vi "Process each eye.vi"(0 "Camera coordinates rel to head co-ordinates":T1 {"y" format="%.2f"; "z" format="%.2f"; "theta" format="%.2f"; "phi" format="%.2f"; "d" format="%.2f"}, 1 "Time (sec)":sgl[](array[numeric]) format="%.4f", 2 "Dir":enum16{"Right", "Left"}(ring), 3 "Hor (F)":dbl[](array[numeric]) format="%.2f", 4 "Ver (F)":dbl[](array[numeric]) format="%.2f", 5 "Posn, Vel, Acc 2":dbl[][](array[numeric]), 6 "Angles":bool, 7 "Point1":dbl[][](array[numeric]) format="%.2f", 8 "Trigger Edge":i32, 9 "Tor (F)":dbl[](array[numeric]) format="%.2f", 10 "Position Convention":u16(ring) items=["Fick Angles", "Rotation Vectors"], 11 "Point2":dbl[][](array[numeric]) format="%.2f", 12 "Sample Rate":i32, 13 "Point3":dbl[][](array[numeric]) format="%.2f", 16 "Savol Filter in percent":dbl=3.0 format="%#_13g", 18 "Use Last":bool, 19 "VOG system":enum16{"Mouse", "Chinchilla"}(ring)) -> (14 "Posn, Vel, Acc":dbl[][](array[numeric]) format="%.2f", 17 "cancelled":bool)   [LabVIEW 2016, in "3 dot tracker.lvlib"]
uses:
  3 dot tracker.lvlib
  <vilib>/Analysis/3filter.llb/Savitzky-Golay Filter (DBL).vi
  <vilib>/Analysis/baseanly.llb/A x Vector.vi
  comm/fick-matrix/fick-matrix.lvlib
  <vilib>/Analysis/NI_AALBase.lvlib
  comm/quaternion/quaternion.lvlib
  <vilib>/ptbypt/NI_PtbyPt.lvlib
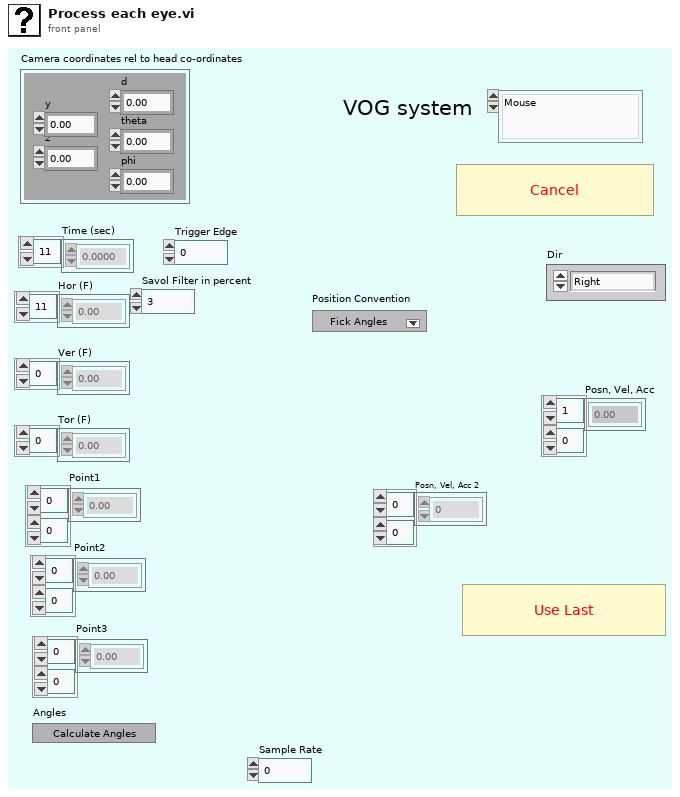
[diagram p1: front panel]
types:
  T1 = cluster{"d":dbl, "phi":dbl, "theta":dbl, "z":dbl, "y":dbl}
  T2 = cluster{"Point1":dbl[], "Point2":dbl[], "Point3":dbl[]}
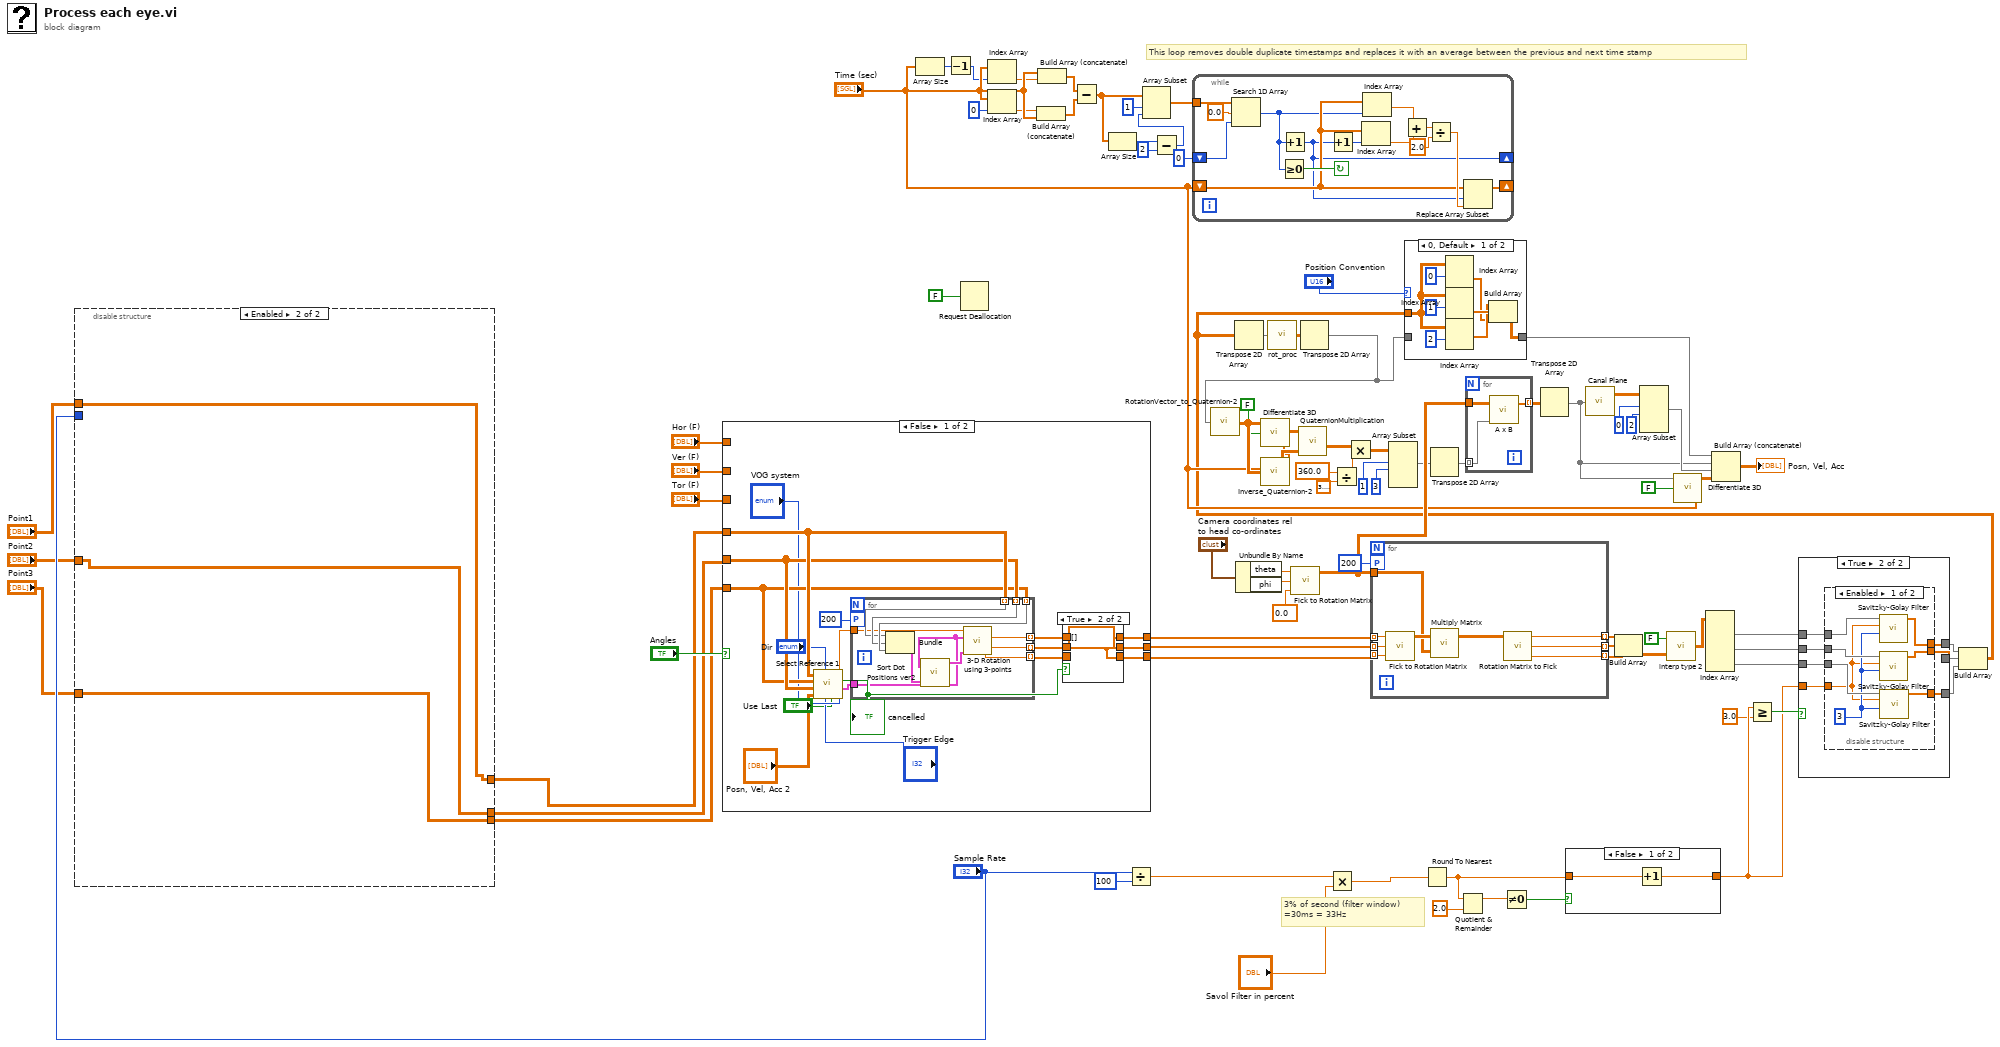
[diagram p0: block diagram]
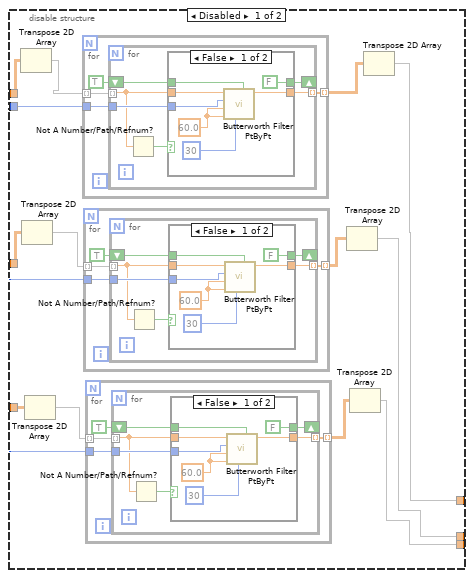
[diagram p2: hidden frame]
diagram:
  # "3% of second (filter window)\n=30ms = 33Hz"
  # "This loop removes double duplicate timestamps and replaces it with an average between the previous and next time stamp"
  n1 = disable-structure shown="Enabled" {
    disable-tunnel: "Sample Rate" -> [w100 _]
    disable-tunnel: "Point1" -> [w99 w160]
    disable-tunnel: [w96 w160] -> w5
    disable-tunnel: [w94 w158] -> w4
    disable-tunnel: [w93 w159] -> w3
    disable-tunnel: "Point2" -> [w90 w159]
    disable-tunnel: "Point3" -> [w89 w158]
    frame Disabled {
      n2 = Transpose 2D Array(2D array=w99) -> (transposed array=w98:dbl[][])
      n3 = Transpose 2D Array(2D array=w90) -> (transposed array=w91:dbl[][])
      n4 = Transpose 2D Array(2D array=w89) -> (transposed array=w88:dbl[][])
      n5 = for {
        tunnel: w98 -> [w142] mode=indexing
        tunnel: w100 -> [w141]
        tunnel: [w139] -> w97 mode=indexing
        n6 = for {
          tunnel: w142 -> [w145] mode=indexing
          tunnel: w141 -> [w148]
          shift-right: [w143] -> _
          shift-left: TRUE -> [w147]
          tunnel: [w144] -> w139 mode=indexing
          n7 = Not A Number/Path/Refnum?(number/path/refnum=w145) -> (NaN/Path/Refnum?=w146:bool)
          n8 = case shown="False" w146 {
            tunnel: w145 -> [w150 w157]
            tunnel: w148 -> [w155 _]
            tunnel: w147 -> [w152 w156]
            tunnel: [w153 w157] -> w144
            tunnel: [FALSE w156] -> w143
            frame False {
              w154 = 60.0 ("high cutoff freq: fh")
              n9 = call <vilib>:"Butterworth Filter PtByPt.vi"("initialize"=w152, "order"=30, "low cutoff freq: fl"=w154, "high cutoff freq: fh"=w154, "sampling freq: fs"=w155, "x"=w150) -> ("Filtered x"=w153:dbl)  [unwired: 3 in, 1 out]
            }
            frame True {
            }
          }
        }
      }
      n10 = for {
        tunnel: w91 -> [w123] mode=indexing
        tunnel: w100 -> [w122]
        tunnel: [w120] -> w92 mode=indexing
        n11 = for {
          tunnel: w123 -> [w126] mode=indexing
          tunnel: w122 -> [w129]
          shift-right: [w124] -> _
          shift-left: TRUE -> [w128]
          tunnel: [w125] -> w120 mode=indexing
          n12 = Not A Number/Path/Refnum?(number/path/refnum=w126) -> (NaN/Path/Refnum?=w127:bool)
          n13 = case shown="False" w127 {
            tunnel: w126 -> [w131 w138]
            tunnel: w129 -> [w136 _]
            tunnel: w128 -> [w133 w137]
            tunnel: [w134 w138] -> w125
            tunnel: [FALSE w137] -> w124
            frame False {
              w135 = 60.0 ("high cutoff freq: fh")
              n14 = call <vilib>:"Butterworth Filter PtByPt.vi"("initialize"=w133, "order"=30, "low cutoff freq: fl"=w135, "high cutoff freq: fh"=w135, "sampling freq: fs"=w136, "x"=w131) -> ("Filtered x"=w134:dbl)  [unwired: 3 in, 1 out]
            }
            frame True {
            }
          }
        }
      }
      n15 = for {
        tunnel: w88 -> [w104] mode=indexing
        tunnel: w100 -> [w103]
        tunnel: [w101] -> w95 mode=indexing
        n16 = for {
          tunnel: w104 -> [w107] mode=indexing
          tunnel: w103 -> [w110]
          shift-right: [w105] -> _
          shift-left: TRUE -> [w109]
          tunnel: [w106] -> w101 mode=indexing
          n17 = Not A Number/Path/Refnum?(number/path/refnum=w107) -> (NaN/Path/Refnum?=w108:bool)
          n18 = case shown="False" w108 {
            tunnel: w107 -> [w112 w119]
            tunnel: w110 -> [w117 _]
            tunnel: w109 -> [w114 w118]
            tunnel: [w115 w119] -> w106
            tunnel: [FALSE w118] -> w105
            frame False {
              w116 = 60.0 ("high cutoff freq: fh")
              n19 = call <vilib>:"Butterworth Filter PtByPt.vi"("initialize"=w114, "order"=30, "low cutoff freq: fl"=w116, "high cutoff freq: fh"=w116, "sampling freq: fs"=w117, "x"=w112) -> ("Filtered x"=w115:dbl)  [unwired: 3 in, 1 out]
            }
            frame True {
            }
          }
        }
      }
      n20 = Transpose 2D Array(2D array=w92) -> (transposed array=w93:dbl[][])
      n21 = Transpose 2D Array(2D array=w95) -> (transposed array=w94:dbl[][])
      n22 = Transpose 2D Array(2D array=w97) -> (transposed array=w96:dbl[][])
    }
    frame Enabled {
    }
  }
  n23 = case shown="False" "Angles" {
    tunnel: [w169 w195] -> w15
    tunnel: [w168 w194] -> w17
    tunnel: [w167 w193] -> w16
    tunnel: "Hor (F)" -> [_ w195]
    tunnel: "Ver (F)" -> [_ w194]
    tunnel: "Tor (F)" -> [_ w193]
    tunnel: w5 -> [w176 _]
    tunnel: w3 -> [w175 _]
    tunnel: w4 -> [w174 _]
    frame False {
      n24 = call "Select Reference 1.vi"("VOG system"="VOG system", "Use Last"="Use Last", "Trigger Edge"="Trigger Edge", "Dir"="Dir", "Posn, Vel, Acc"="Posn, Vel, Acc 2", "Point2"=w175, "Point3"=w174, "Point1"=w176) -> ("Pupil Baseline Info"=w178:T2, "cancelled"=w166:bool, "Radius of eyeball (pixels)"=w177:dbl)  [unwired: 1 in]
      "cancelled" <- w166
      n25 = for {
        tunnel: w174 -> [w192] mode=indexing
        tunnel: w175 -> [w191] mode=indexing
        tunnel: w176 -> [w190] mode=indexing
        tunnel: w177 -> [w189]
        tunnel: [w188] -> w165 mode=indexing
        tunnel: [w187] -> w164 mode=indexing
        tunnel: [w186] -> w163 mode=indexing
        tunnel: w178 -> [w183]
        workers-P: 200 -> [_]
        n26 = Bundle("Point1"=w190, "Point2"=w191, "Point3"=w192) -> (w185:T2)  [unwired: 1 in]
        n27 = call "Sort Dot Positions ver2.vi"("Present Position (input)"=w185, "Previous Position"=w183) -> ("Present Position (output)"=w184:T2)
        n28 = call "3-D Rotation using 3-points.vi"("Present Position"=w184, "Initial Position"=w183, "Radius of eyeball in pixels"=w189) -> ("T"=w186:dbl, "V"=w187:dbl, "H"=w188:dbl)  [unwired: 1 in, 1 out]
      }
      n29 = case shown="True" w166 {
        tunnel: [w181 w182] -> w169
        tunnel: [w180 w182] -> w168
        tunnel: [w179 w182] -> w167
        tunnel: w165 -> [w181 _]
        tunnel: w164 -> [w180 _]
        tunnel: w163 -> [w179 _]
        frame False {
        }
        frame True {
          w182 = dbl[] []
        }
      }
    }
    frame True {
    }
  }
  n30 = Array Size(array="Time (sec)") -> (size(s)=w49:i32)
  n31 = Decrement(x=w49) -> (x-1=w43:i32)
  n32 = Request Deallocation(FALSE ("flag")) -> ()
  n33 = Index Array(array="Time (sec)", index=w43) -> (element=w47:sgl)
  n34 = Index Array(array="Time (sec)", index=0) -> (element=w46:sgl)
  n35 = Build Array (concatenate)(w46, "Time (sec)") -> (w44:sgl[])
  n36 = Build Array (concatenate)("Time (sec)", w47) -> (w45:sgl[])
  n37 = Subtract(x=w45, y=w44) -> (x-y=w41:sgl[])
  n38 = Array Size(array=w41) -> (size(s)=w40:i32)
  n39 = Divide(x="Sample Rate", y=100) -> (x/y=w19:dbl)
  n40 = Subtract(x=w40, y=2) -> (x-y=w38:i32)
  n41 = Array Subset(array=w41, index=1, length=w38) -> (w37:sgl[])
  n42 = while {
    tunnel: w37 -> [w209]
    shift-right: [w197] -> _
    shift-left: 0 ("index of element") -> [w206]
    shift-right: [w198] -> _
    shift-left: "Time (sec)" -> [w199]
    stop <- w207 continue-if-true
    n43 = Search 1D Array(1D array=w209, element=0.0, start index (0)=w206) -> (index of element=w196:i32)
    n44 = Greater Or Equal To 0?(x=w196) -> (x >= 0?=w207:bool)
    n45 = Increment(x=w196) -> (x+1=w197:i32)
    n46 = Increment(x=w197) -> (x+1=w205:i32)
    n47 = Index Array(array=w199, index=w205) -> (element=w204:sgl)
    n48 = Index Array(array=w199, index=w196) -> (element=w203:sgl)
    n49 = Add(x=w203, y=w204) -> (x+y=w202:sgl)
    n50 = Divide(x=w202, y=2.0) -> (x/y=w200:dbl)
    n51 = Replace Array Subset(array=w199, new element=w200, index=w197) -> (w198:sgl[])
  }
  n52 = Unbundle By Name("Camera coordinates rel to head co-ordinates") -> ("theta"=w65:dbl, "phi"=w64:dbl)
  n53 = call "Fick to Rotation Matrix.vi"("T"=0.0, "V"=w64, "H"=w65) -> ("Rotation Matrix"=w56:dbl[][])
  n54 = Multiply(x=w19, y="Savol Filter in percent") -> (x*y=w20:dbl)
  n55 = Divide(x=360.0, y=3.141592653589793) -> (x/y=w81:dbl)
  n56 = for {
    tunnel: w16 -> [w216] mode=indexing
    tunnel: w17 -> [w217] mode=indexing
    tunnel: w15 -> [w218] mode=indexing
    tunnel: [w214] -> w34 mode=indexing
    tunnel: [w213] -> w33 mode=indexing
    tunnel: [w212] -> w32 mode=indexing
    tunnel: w56 -> [w210]
    workers-P: 200 -> [_]
    n57 = call "Fick to Rotation Matrix.vi"("T"=w216, "V"=w217, "H"=w218) -> ("Rotation Matrix"=w215:dbl[][])
    n58 = call "Multiply Matrix.vi"("1st rotation Matrix"=w210, "2nd rotation Matrix"=w215) -> ("Resultant Matrix"=w211:dbl[][])  [unwired: 1 in]
    n59 = call "Rotation Matrix to Fick.vi"("A"=w211) -> ("T"=w212:dbl, "V"=w213:dbl, "H"=w214:dbl)  [unwired: 2 in]
  }
  n60 = Round To Nearest(number=w20) -> (nearest integer value=w21:dbl)
  n61 = Quotient & Remainder(x=w21, y=2.0) -> (x-y*floor(x/y)=w23:dbl)  [unwired: 1 out]
  n62 = Not Equal To 0?(x=w23) -> (x != 0?=w22:bool)
  n63 = case shown="False" w22 {
    tunnel: w21 -> [w220 w221]
    tunnel: [w219 w221] -> w10
    frame False {
      n64 = Increment(x=w220) -> (x+1=w219:dbl)
    }
    frame True {
    }
  }
  n65 = Build Array(w34, w33, w32) -> (w35:dbl[][])
  n66 = call "interp type 2.vi"("NaN"=w35, "Remove front and end"=FALSE) -> ("Interpolated"=w31:dbl[][])
  n67 = Index Array(array=w31) -> (element #1=w14:dbl[], element #2=w13:dbl[], element #3=w12:dbl[])  [unwired: 6 in]
  n68 = Greater Or Equal?(x=w10, y=3.0) -> (x >= y?=w11:bool)
  n69 = case shown="True" w11 {
    tunnel: [w224 w231] -> w30
    tunnel: [w223 w230] -> w29
    tunnel: [w222 w229] -> w28
    tunnel: w10 -> [_ w228]
    tunnel: w14 -> [w224 w227]
    tunnel: w13 -> [w223 w226]
    tunnel: w12 -> [w222 w225]
    frame False {
    }
    frame True {
      n70 = disable-structure shown="Enabled" {
        disable-tunnel: w227 -> [w239 w242]
        disable-tunnel: [w238 w242] -> w231
        disable-tunnel: w226 -> [w237 w241]
        disable-tunnel: [w236 w241] -> w230
        disable-tunnel: w225 -> [w235 w240]
        disable-tunnel: [w234 w240] -> w229
        disable-tunnel: w228 -> [w232 _]
        frame Enabled {
          w233 = 3 ("polynomial order")
          n71 = call-poly <vilib>:"Savitzky-Golay Filter.vi"("polynomial order"=w233, "side points"=w232, "X"=w239) -> ("Filtered X"=w238:dbl[])  [unwired: 7 in, 1 out]
          n72 = call-poly <vilib>:"Savitzky-Golay Filter.vi"("polynomial order"=w233, "side points"=w232, "X"=w237) -> ("Filtered X"=w236:dbl[])  [unwired: 7 in, 1 out]
          n73 = call-poly <vilib>:"Savitzky-Golay Filter.vi"("polynomial order"=w233, "side points"=w232, "X"=w235) -> ("Filtered X"=w234:dbl[])  [unwired: 7 in, 1 out]
        }
        frame Disabled {
        }
      }
    }
  }
  n74 = Build Array(w30, w29, w28) -> (w27:dbl[][])
  n75 = Transpose 2D Array(2D array=w27) -> (transposed array=w68:dbl[][])
  n76 = call "rot_proc.vi"("Euler Angles"=w68) -> ("Rotation Vectors"=w69:dbl[][])  [unwired: 17 in, 1 out]
  n77 = Transpose 2D Array(2D array=w69) -> (transposed array=w58:dbl[][])
  n78 = call "RotationVector_to_Quaternion-2.vi"("rotation vectors"=w58) -> ("quaternions"=w77:dbl[][])  [unwired: 4 in]
  n79 = call "Differentiate 3D.vi"("Timebase"="Time (sec)", "Fixed Sample Rate"=FALSE, "Data (in)"=w77) -> ("Data (differentiated)"=w86:dbl[][])  [unwired: 2 in]
  n80 = call "Inverse_Quaternion-2.vi"("quaternions"=w77) -> ("inverse quaternions"=w85:dbl[][])  [unwired: 4 in]
  n81 = call "QuaternionMultiplication.vi"("quaternions B"=w85, "quaternions A"=w86) -> ("quaternions A x B"=w84:dbl[][])  [unwired: 3 in]
  n82 = Multiply(x=w84, y=w81) -> (x*y=w70:dbl[][])
  n83 = Array Subset(array=w70, index (row)=1 ("Array Index"), length (row)=3 ("Array Index")) -> (w54:dbl[][])  [unwired: 2 in]
  n84 = case shown="0, Default" "Position Convention" {
    tunnel: w27 -> [w250 _]
    tunnel: w58 -> [_ w251]
    tunnel: [w243 w251] -> w59
    frame 0, Default {
      n85 = Index Array(array=w250, index (row)=0) -> (element=w244:dbl[])  [unwired: 1 in]
      n86 = Index Array(array=w250, index (row)=1) -> (element=w246:dbl[])  [unwired: 1 in]
      n87 = Index Array(array=w250, index (row)=2) -> (element=w245:dbl[])  [unwired: 1 in]
      n88 = Build Array(w245, w246, w244) -> (w243:dbl[][])
    }
    frame 1 {
    }
  }
  n89 = Transpose 2D Array(2D array=w54) -> (transposed array=w53:dbl[][])
  n90 = for {
    tunnel: w53 -> [w253] mode=indexing
    tunnel: w56 -> [w254]
    tunnel: [w252] -> w55 mode=indexing
    n91 = call-poly <vilib>:"A x B.vi"("Vector"=w253, "A"=w254) -> ("A x Vector"=w252:dbl[])  [unwired: 1 out]
  }
  n92 = Transpose 2D Array(2D array=w55) -> (transposed array=w52:dbl[][])
  n93 = call "Canal Plane.vi"("Principal Planes"=w52) -> ("Canal Planes"=w80:dbl[][])
  n94 = Array Subset(array=w80, index (row)=0 ("Array Index"), length (row)=2 ("Array Index")) -> (w74:dbl[][])  [unwired: 2 in]
  n95 = call "Differentiate 3D.vi"("Timebase"="Time (sec)", "Fixed Sample Rate"=FALSE, "Data (in)"=w52) -> ("Data (differentiated)"=w73:dbl[][])  [unwired: 2 in]
  n96 = Build Array (concatenate)(w59, w52, w74, w73) -> (→"Posn, Vel, Acc":dbl[][])
